vi "Insert Halt.vi"(8 "error in (no error)":errorcluster, 10 "Insert Halt":T1, 11 "Test Executive Builder Model in":refnum<class "Test Executive Builder Model.lvclass">) -> (0 "error out":errorcluster, 3 "Test Executive Builder Model out":refnum<class "Test Executive Builder Model.lvclass">, 5 "Unique ID out":string)   [LabVIEW 2019, in "Test Executive Builder Model.lvclass"]
uses:
  <vilib>/gpm_packages/@cs/Test-executive-builder/Source/Test Executive Builder Model/Test Executive Builder Model/Test Executive Builder Model.lvclass
  C:/Program Files/National Instruments/LabVIEW 2019/vi.lib/ActorFramework/Actor/Actor.lvclass
  <vilib>/gpm_packages/@cs/Test-executive-builder/Source/Application Dependencies/Insert Halt.ctl
  <vilib>/gpm_packages/@cs/Test-executive-builder/Source/Test Executive Builder Model/Test Executive Builder Model/Test Executive Builder Model.lvclass/Test Executive Builder Model.ctl
  <vilib>/ActorFramework/Actor/Actor.lvclass/Actor.ctl
  <vilib>/ActorFramework/Message Enqueuer/Message Enqueuer.lvclass/Message Enqueuer.ctl
  <vilib>/ActorFramework/Message Enqueuer/Init from Existing Queue.vi
  <vilib>/ActorFramework/Message Enqueuer/Enqueue.vi
  <vilib>/gpm_packages/@cs/Test-executive-builder/Source/Test Executive Builder Model/Test Executive Builder Model Messages/Redraw Tree Msg/Redraw Tree Msg.lvclass
  C:/Program Files/National Instruments/LabVIEW 2019/vi.lib/ActorFramework/Message/Message.lvclass
  <vilib>/ActorFramework/Message Priority Queue/Priority Enqueue.vi
  <vilib>/ActorFramework/Message Enqueuer/Message Enqueuer.lvclass
  <vilib>/ActorFramework/Actor/Actor.lvclass
  <vilib>/gpm_packages/@cs/test-executive/Source/Test Executive/TestExecutive Ref/TestExecutive Ref.lvclass
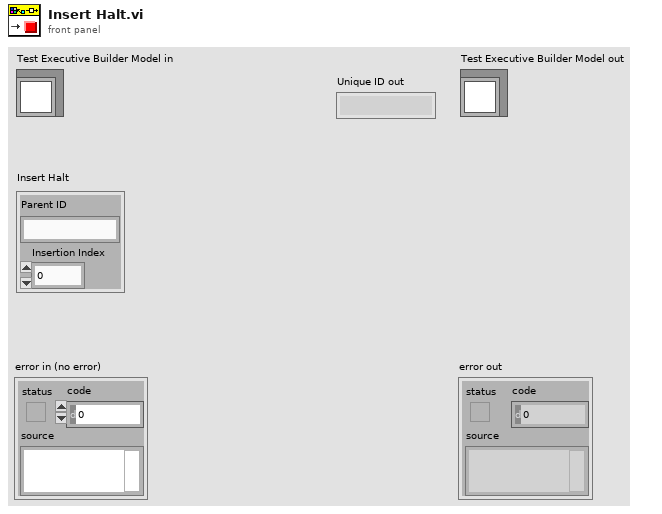
[diagram p1: front panel]
types:
  T1 = typedef "Insert Halt.ctl" = cluster{"Parent ID":string, "Insertion Index":i32}
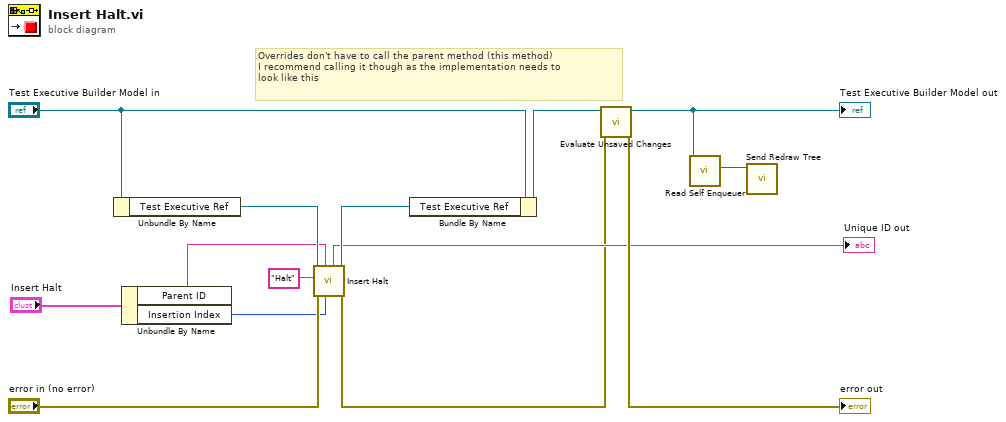
[diagram p0: block diagram]
diagram:
  # "Overrides don't have to call the parent method (this method)\nI recommend calling it though as the implementation needs to\nlook like this"
  n1 = Unbundle By Name("Test Executive Builder Model in") -> ("Test Executive Ref"=w8:refnum<data-value>)
  n2 = Unbundle By Name("Insert Halt") -> ("Parent ID"=w6:string, "Insertion Index"=w2:i32)
  n3 = call <vilib>:"Insert Halt.vi"("Insertion Index"=w2, "Parent ID"=w6, "error in (no error)"="error in (no error)", "Name"="Halt", "Test Executive Ref"=w8) -> ("error out"=w3:errorcluster, "Test Executive Ref out"=w7:refnum<data-value>, "Unique ID out"=→"Unique ID out":string)  [unwired: 3 in, 1 out]
  n4 = Bundle By Name(cluster="Test Executive Builder Model in", "Test Executive Ref"=w7) -> (w12:refnum<class "Test Executive Builder Model.lvclass">)
  n5 = call-dynamic "Evaluate Unsaved Changes.vi"("error in (no error)"=w3, "Test Executive Builder Model in"=w12) -> ("error out"=→"error out":errorcluster, "Test Executive Builder Model out"=w11:refnum<class "Test Executive Builder Model.lvclass">)  [unwired: 8 in]
  "Test Executive Builder Model out" <- w11
  n6 = call <vilib>:"Read Self Enqueuer.vi"("Actor"=w11) -> ("Self Enqueuer"=w13:refnum<class "Message Enqueuer.lvclass">)  [unwired: 10 in]
  n7 = call <vilib>:"Send Redraw Tree.vi"("Message Enqueuer"=w13) -> ()  [unwired: 9 in, 2 out]
